vi "Deregister FKs.vi"(8 "error in (no error)":errorcluster, 10 "Form ID":T1, 11 "Form Server in":refnum<class "Form Server.lvclass">) -> (0 "error out":errorcluster, 3 "Form Server out":refnum<class "Form Server.lvclass">)   [LabVIEW 2020, in "Form Server.lvlib" / "Form Server.lvclass"]
uses:
  Form Server.lvclass
  Autoclose manager/Form ID.ctl
  Form Server.lvclass/Form Server.ctl
  Form Server Configuration/Form Server Configuration.lvclass/Form Server Configuration.ctl
  Update Fields Logic/Update Fields Logic.lvclass
  Form Server Configuration/Form Server Configuration.lvclass
  Form Server Interfaces.lvlib
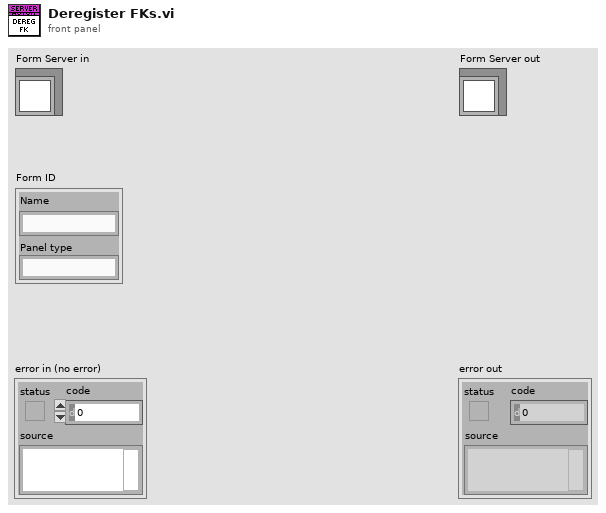
[diagram p1: front panel]
types:
  T1 = typedef "Form Server Interfaces.lvlib/Form ID.ctl" = cluster{"Name":string, "Panel type":string}
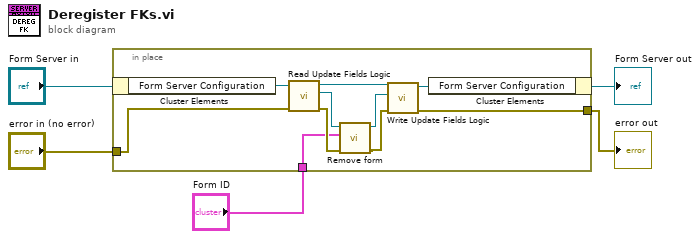
[diagram p0: block diagram]
diagram:
  n1 = in-place {
    in-place-border: [w12] -> w3
    in-place-border: "error in (no error)" -> [w11]
    in-place-border: "Form ID" -> [w6]
    n2 = in-place-cluster #1("Form Server in") -> ("Form Server Configuration"=w15:refnum<class "Form Server Configuration.lvclass">)
    n3 = call "Read Update Fields Logic.vi"("error in (no error)"=w11, "Form Server Configuration in"=w15) -> ("error out"=w7:errorcluster, "Form Server Interfaces.lvlib:Update Fields Logic.lvclass"=w10:refnum<class "Update Fields Logic.lvclass">, "Form Server Configuration out"=w14:refnum<class "Form Server Configuration.lvclass">)  [unwired: 7 in]
    n4 = call-dynamic "Remove form.vi"("error in (no error)"=w7, "Form ID"=w6, "Update Fields Logic in"=w10) -> ("error out"=w8:errorcluster, "Update Fields Logic out"=w9:refnum<class "Update Fields Logic.lvclass">)  [unwired: 7 in]
    n5 = call "Write Update Fields Logic.vi"("error in (no error)"=w8, "Form Server Interfaces.lvlib:Update Fields Logic.lvclass"=w9, "Form Server Configuration in"=w14) -> ("error out"=w12:errorcluster, "Form Server Configuration out"=w13:refnum<class "Form Server Configuration.lvclass">)  [unwired: 7 in]
    n6 = in-place-cluster #1("Form Server Configuration"=w13) -> (→"Form Server out":refnum<class "Form Server.lvclass">)
  }
  "error out" <- w3
